vi "GetWebcams.vi"() -> ()   [LabVIEW 2021]
doc: "This VI retrieves JPEGs from URLs specified in Webcams.ini, in the rig's \"All_Users\" folder. It applies overlay text, if required, and saves the image(s) to the Pictures folder, with a name based on the RawData file name."
uses:
  Anemometry/Anemometry Sub Vis/Globals/Meas_global.vi
  Anemometry/Anemometry Sub Vis/Globals/Constants_global.vi
panel:
  out "Overlay Text":string
  # "This VI retrieves JPEGs from URLs specified in Webcams.ini, in the rig's \"All_Users\" folder. It applies overlay text, obtained from MeasurementGlobal, if required, and saves the image(s) to the Pictures folder, with a name based on the RawData file name."
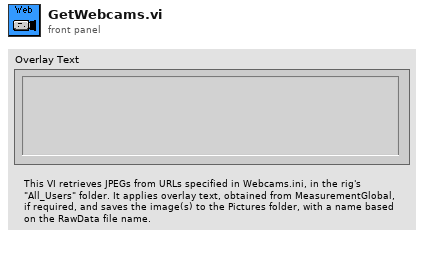
[diagram p1: front panel]
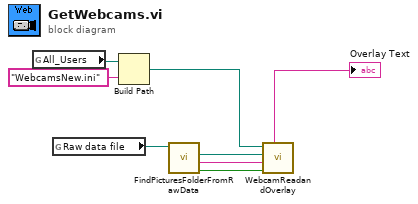
[diagram p0: block diagram]
diagram:
  n1 = global read "Constants_global.vi" "All_Users"() -> (w8:path)
  n2 = global read "Meas_global.vi" "Raw data file"() -> (w5:path)
  n3 = Build Path(base path=w8, name or relative path="WebcamsNew.ini") -> (appended path=w7:path)
  n4 = call "FindPicturesFolderFromRawData.vi"("RawDataFile"=w5) -> ("SurreyPath?"=w1:bool, "RawDataName"=w3:string, "PicturesPath"=w4:path)  [unwired: 8 in]
  n5 = call "WebcamReadandOverlay.vi"("SurreyPath?"=w1, "BaseName"=w3, "BasePathToSaveTo"=w4, "WebcamFilePath"=w7) -> ("OverlayText"=→"Overlay Text":string)  [unwired: 6 in, 1 out]
